vi "ControlSolenoidTurnOn.vi"(2 "On?":bool) -> (0 "error out":errorcluster, 1 "task out":refnum<k21>)   [LabVIEW 2014]
uses:
  <vilib>/DAQmx/write.llb/DAQmx Write (Digital 1D Bool NChan 1Samp 1Line).vi
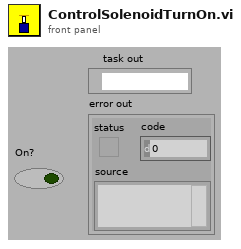
[diagram p1: front panel]
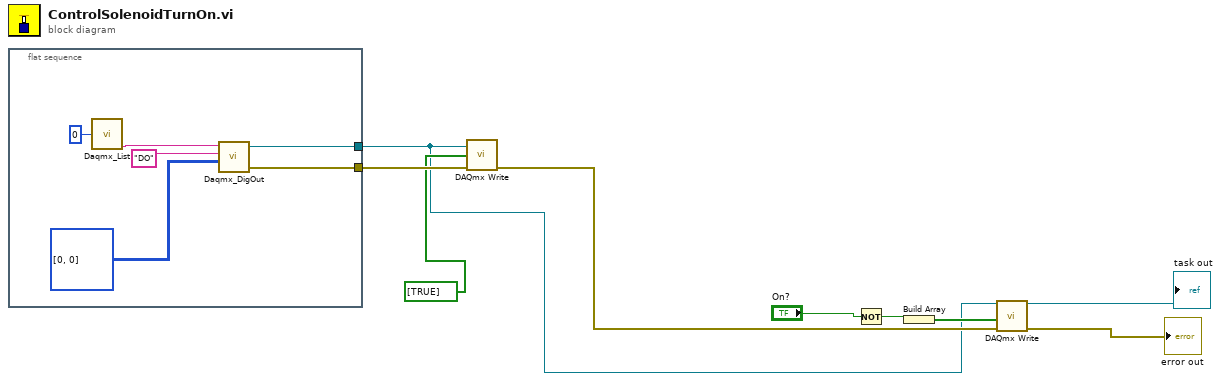
[diagram p0: block diagram]
diagram:
  n1 = flat-sequence {
    tunnel: [w11] -> w9
    tunnel: [w12] -> w3
    frame #0 {
      n2 = call "Daqmx_List.vi"("Device Number n"=u8 0) -> ("NI-DAQmx Device Name n"=w13:tag)  [unwired: 3 out]
      n3 = call "Daqmx_DigOut.vi"("Array of Ports, Lines"=u8[][] [[0, 0]], "Base Task Name"="DO", "DAQmx device name"=w13) -> ("error out"=w11:errorcluster, "Output Task Name"=w12:refnum<k21>)  [unwired: 1 in, 1 out]
    }
  }
  n4 = call-poly <vilib>:"DAQmx Write.vi"("task/channels in"=w3, "data"=bool[] [TRUE], "error in"=w9) -> ("error out"=w4:errorcluster)  [unwired: 1 in, 11 out]
  n5 = Not(x="On?") -> (.not. x?=w6:bool)
  n6 = Build Array(w6) -> (w7:bool[])
  n7 = call-poly <vilib>:"DAQmx Write.vi"("task/channels in"=w3, "data"=w7, "error in"=w4) -> ("task out"=→"task out":refnum<k21>, "error out"=→"error out":errorcluster)  [unwired: 1 in, 10 out]
